vi "PCAN_DecompMessage.vi"(11 "CAN_Message out":T1) -> (0 "Intensity (a.u.)":dbl, 1 "Detector2 Shutter Open?":bool, 2 "Detector1 Shutter Open?":bool, 3 "Excitation Shutter Open?":bool)   [LabVIEW 8.6]
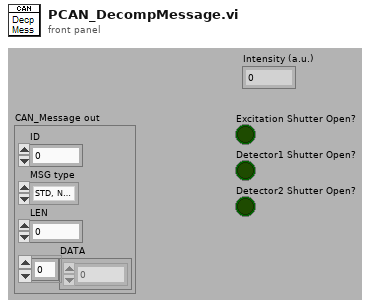
[diagram p1: front panel]
types:
  T1 = cluster{"ID":u32, "MSG type":enum8{"STD, NO RTR", "STD,RTR", "XTD, NO RTR", "XTD, RTR"}, "LEN":u8, "DATA":u8[]}
  T2 = enum8{"STD, NO RTR", "STD,RTR", "XTD, NO RTR", "XTD, RTR"}
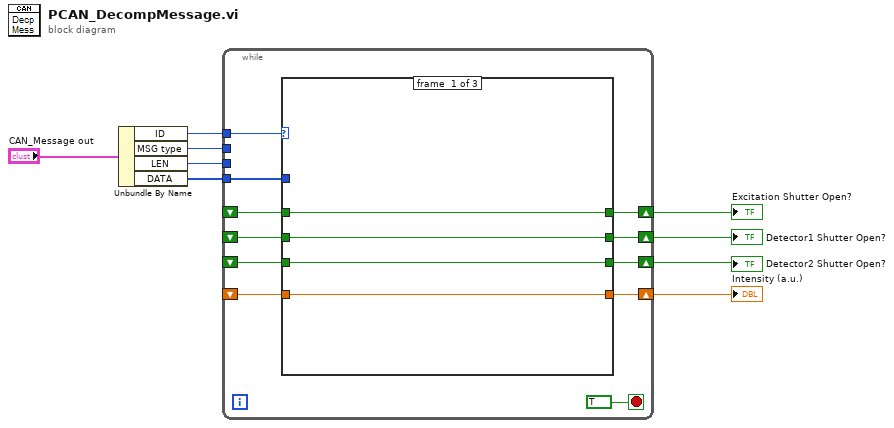
[diagram p0: block diagram]
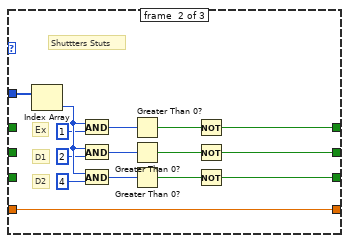
[diagram p2: hidden frame]
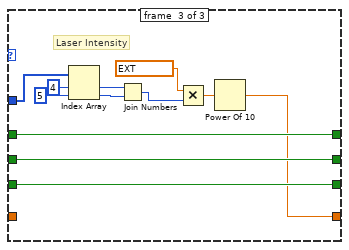
[diagram p3: hidden frame]
diagram:
  n1 = Unbundle By Name("CAN_Message out") -> ("ID"=w8:u32, "MSG type"=w7:T2, "LEN"=w6:u8, "DATA"=w5:u8[])
  n2 = while {
    tunnel: w8 -> [w19]
    tunnel: w7 -> [_]
    tunnel: w6 -> [_]
    tunnel: w5 -> [w18]
    shift-right: [w17] -> w3
    shift-left: _ -> [w12]
    shift-right: [w16] -> w2
    shift-left: _ -> [w13]
    shift-right: [w15] -> w4
    shift-left: _ -> [w14]
    shift-right: [w11] -> w1
    shift-left: _ -> [w10]
    stop <- TRUE stop-if-true
    n3 = case shown="257" w19 {
      tunnel: w18 -> [_ w39 w48]
      tunnel: [w22 w28 w49] -> w17
      tunnel: [w23 w27 w50] -> w16
      tunnel: [w24 w26 w51] -> w15
      tunnel: w14 -> [w24 _ w51]
      tunnel: w13 -> [w23 _ w50]
      tunnel: w12 -> [w22 _ w49]
      tunnel: [w21 w25 w41] -> w11
      tunnel: w10 -> [w21 w25 _]
      frame #0 {
      }
      frame #1 {
        # "Shuttters Stuts"
        # "D2"
        # "D1"
        # "Ex"
        n4 = Index Array(array=w39) -> (element=w38:u8)  [unwired: 1 in]
        n5 = And(x=w38, y=u8 1) -> (x .and. y?=w34:u8)
        n6 = And(x=w38, y=u8 2) -> (x .and. y?=w33:u8)
        n7 = And(x=w38, y=u8 4) -> (x .and. y?=w32:u8)
        n8 = Greater Than 0?(x=w34) -> (x > 0?=w31:bool)
        n9 = Greater Than 0?(x=w33) -> (x > 0?=w30:bool)
        n10 = Greater Than 0?(x=w32) -> (x > 0?=w29:bool)
        n11 = Not(x=w31) -> (.not. x?=w26:bool)
        n12 = Not(x=w30) -> (.not. x?=w27:bool)
        n13 = Not(x=w29) -> (.not. x?=w28:bool)
      }
      frame #2 {
        # "Laser Intensity"
        n14 = Index Array(array=w48, index #1=4 ("index"), index #2=5 ("index")) -> (element #1=w45:u8, element #2=w44:u8)
        n15 = Join Numbers(hi=w45, lo=w44) -> ((hi.lo)=w40:u16)
        n16 = Multiply(x=ext 0.0097752, y=w40) -> (x*y=w42:ext)
        n17 = Power Of 10(x=w42) -> (10^x=w41:ext)
      }
    }
  }
  "Excitation Shutter Open?" <- w4
  "Detector2 Shutter Open?" <- w3
  "Detector1 Shutter Open?" <- w2
  "Intensity (a.u.)" <- w1
